vi "MetersToPixels.vi"(10 "meters":dbl) -> (2 "pixels":i32)   [LabVIEW 2009, in "Host.lvlib" / "Draw.lvlib"]
uses:
  Draw.lvlib
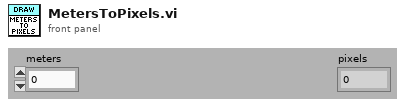
[diagram p1: front panel]
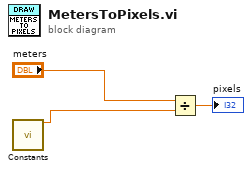
[diagram p0: block diagram]
diagram:
  n1 = call "Constants.vi"() -> ("MetersInPixel"=w3:dbl)  [unwired: 16 in, 3 out]
  n2 = Divide(x="meters", y=w3) -> (x/y=→"pixels":dbl)
